vi "niRFUtil LCAPI Copy 1D Array (1 SGL).vi"(0 "Source0 1D Array (SGL)":sgl[](array[numeric]) format="%.2f", 11 "error in (no error)":errorcluster, 12 "Data Copy Descriptor":u64) -> (4 "Source0 Out":sgl[](array[numeric]) format="%.2f", 15 "error out":errorcluster)   [LabVIEW 2015, in "niRFUtil.lvlib"]
uses:
  niRFUtil.lvlib
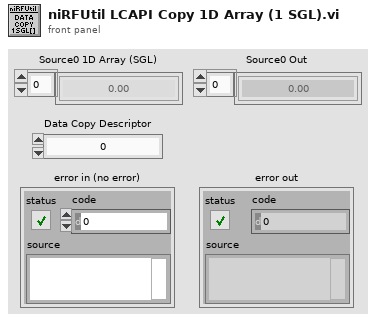
[diagram p1: front panel]
types:
  T1 = cluster{"status":bool, "return type":i32, "errorString":string}
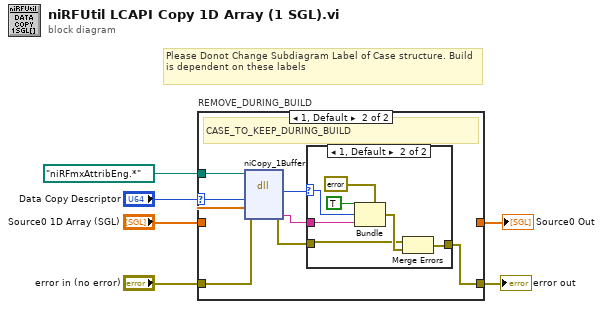
[diagram p0: block diagram]
diagram:
  # "Please Donot Change Subdiagram Label of Case structure. Build is dependent on these labels"
  n1 = case "REMOVE_DURING_BUILD" shown="1, Default" "Data Copy Descriptor" {
    selector: "Data Copy Descriptor" -> [_ w11]
    tunnel: "error in (no error)" -> [w8 w16]
    tunnel: "Source0 1D Array (SGL)" -> [w7 w15]
    tunnel: [w8 w10] -> w3
    tunnel: [w7 _] -> w2
    tunnel: path "niRFmxAttribEng.*" ("path in") -> [_ w9]
    frame 0 {
      # "Development"
    }
    frame 1, Default {
      # "CASE_TO_KEEP_DURING_BUILD"
      n2 = dll-call lib="niRFmxAttribEng.*" fn="niCopy_1Buffer"(path in=w9, error in=w16, "dataCopyDescriptor"=w11, "source0"=w15) -> (error out=w13:errorcluster, "return type"=w14:i32, "errorString"=w12:string)  [unwired: 4 in, 1 out]
      n3 = case shown="1, Default" w14 {
        selector: w14 -> [_ w22]
        tunnel: w12 -> [_ w21]
        tunnel: w13 -> [w17 w19]
        tunnel: [w17 w23] -> w10
        frame 0 {
        }
        frame 1, Default {
          n4 = Bundle(cluster=T1 {"status"=FALSE, "return type"=0, "errorString"=""}, "status"=TRUE, "return type"=w22, "errorString"=w21) -> (w20:T1)
          n5 = Merge Errors(w19, w20) -> (w23:errorcluster)
        }
      }
    }
  }
  "error out" <- w3
  "Source0 Out" <- w2
